vi "User Actor Core Init.vi"(0 "Diplom in":refnum<class "Diplom.lvclass">, 11 "Error in":errorcluster caption="Error in (no error)") -> (4 "Diplom out":refnum<class "Diplom.lvclass">, 15 "Error out":errorcluster)   [LabVIEW 2018, in "HOG Diplom.lvlib" / "Diplom.lvclass"]
doc: "Initialize custom <B>Actor</B> resources. Typical actions:\n\n- Open/create own references.\n- Initialize SW resources.\n- Initialize HW resources.\n- Register additional user events. Beware that external user events are a potential for message racing as those are extra communication channels into <B>Actor</B> that does not follow the message order imposed by the Actor communication tree. If possible convert user event based APIs into message based APIs.\n\n<B>You should not invoke the Call Parent Method node when adding this override.</B>\n\nDefault action\n---------------\nNo action.\n\nSteen Schmidt\nGPower\n2/8 2017"
uses:
  Diplom.lvclass
  C:/Program Files (x86)/National Instruments/LabVIEW 2018/vi.lib/GPower/Actor/Library/Actor Class/Actor.lvclass
  <vilib>/GPower/Actor/Library/Actor Class/Actor.lvclass/Actor.ctl
  Diplom.lvclass/Diplom.ctl
  3a12437a-a909-477d-a8c4-12042c877456.vi
  <vilib>/GPower/Dictionary/Library/Dictionary Class/Get/Get Path.vi
  <vilib>/GPower/Actor/Library/Actor Class/Actor.lvclass
  <vilib>/Utility/NIReport.llb/NI_ReportGenerationCore.lvlib
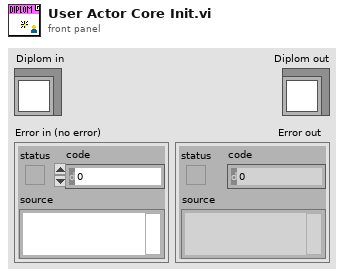
[diagram p1: front panel]
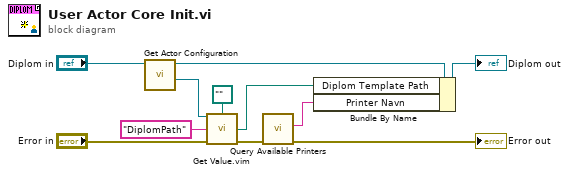
[diagram p0: block diagram]
diagram:
  n1 = call <vilib>:"Get Actor Configuration.vi"("Actor in"="Diplom in") -> ("Actor Configuration"=w8:refnum<class "Dictionary.lvclass">, "Actor out"=w9:refnum<class "Diplom.lvclass">)  [unwired: 9 in]
  n2 = call "Get Value.vim"("Dictionary in"=w8, "Value Type"=path "", "Key Path"="DiplomPath", "Error in"="Error in") -> ("Value"=w5:path, "Error out"=w3:errorcluster)  [unwired: 9 in, 1 out]
  n3 = call <vilib>:"Query Available Printers.vi"("error in (no error)"=w3) -> ("error out"=→"Error out":errorcluster, "default printer"=w1:string)  [unwired: 8 in, 1 out]
  n4 = Bundle By Name(cluster=w9, "Diplom Template Path"=w5, "Printer Navn"=w1) -> (→"Diplom out":refnum<class "Diplom.lvclass">)
